vi "replaceNode.vi"(7 "replaceElementIn":string="/child/son", 8 "error in (no error)":errorcluster, 9 "replaceWithValue":string="Dr C", 11 "SettingsManager in":refnum<class "SettingsManager.lvclass">) -> (0 "error out":errorcluster, 3 "SettingsManager out":refnum<class "SettingsManager.lvclass">)   [LabVIEW 2009, in "Tools.lvlib" / "Settings.lvlib" / "SettingsManager.lvclass"]
uses:
  SettingsManager.lvclass
  SettingsManager.lvclass/SettingsManager.ctl
  xmlNode/xmlNode.lvclass
  XmlParser.lvclass
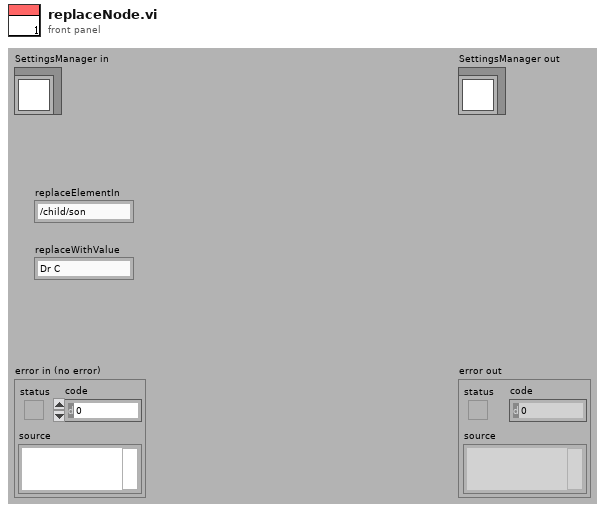
[diagram p1: front panel]
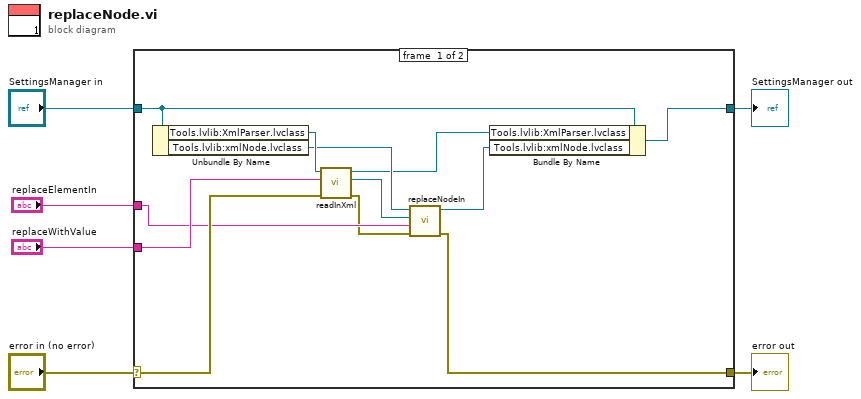
[diagram p0: block diagram]
diagram:
  n1 = case shown="No Error" "error in (no error)" {
    selector: "error in (no error)" -> [w16 w20]
    tunnel: [w8 w20] -> w5
    tunnel: [w7 w19] -> w3
    tunnel: "SettingsManager in" -> [w11 w19]
    tunnel: "replaceWithValue" -> [w17 _]
    tunnel: "replaceElementIn" -> [w13 _]
    frame #0 {
      n2 = Unbundle By Name(w11) -> ("Tools.lvlib:XmlParser.lvclass"=w18:refnum<class "XmlParser.lvclass">, "Tools.lvlib:xmlNode.lvclass"=w15:refnum<class "xmlNode.lvclass">)
      n3 = call "readInXml.vi"("error in (no error)"=w16, "xmlString"=w17, "XmlParser in"=w18) -> ("error out"=w12:errorcluster, "xmlNode"=w14:refnum<class "xmlNode.lvclass">, "XmlParser out"=w10:refnum<class "XmlParser.lvclass">)  [unwired: 6 in]
      n4 = call "replaceNodeIn.vi"("error in (no error)"=w12, "replaceNodeIn"=w13, "xmlNodeReplacement"=w14, "xmlNode in"=w15) -> ("error out"=w8:errorcluster, "xmlNode out"=w9:refnum<class "xmlNode.lvclass">)  [unwired: 6 in]
      n5 = Bundle By Name(cluster=w11, "Tools.lvlib:XmlParser.lvclass"=w10, "Tools.lvlib:xmlNode.lvclass"=w9) -> (w7:refnum<class "SettingsManager.lvclass">)
    }
    frame #1 {
    }
  }
  "error out" <- w5
  "SettingsManager out" <- w3
